vi "M9290A Peak Power.vi"(6 "Reference Level":dbl=20.0, 7 "Route Names":string[](array[string]), 8 "error in":errorcluster, 9 "Span Frequency (50 kHz)":dbl, 10 "Center Frequency (100 MHz)":dbl=1000000000.0, 11 "VISA resource name":refnum<visa-resource-name>="ZVL") -> (0 "error out":errorcluster, 1 "Marker Position":dbl, 2 "Marker Amplitude (Cal)":dbl, 3 "Marker Amplitude (Raw)":dbl)   [LabVIEW 2015]
uses:
  <instrlib>/Agilent MXA Series/Public/Configure/Configure Frequency (Center Span).vi
  <instrlib>/Agilent MXA Series/Public/Configure/Trigger/Configure Trigger (Normal).vi
panel:
  out "VISA resource name out":refnum<visa-resource-name>
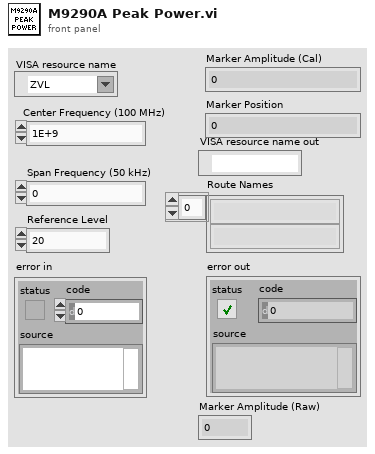
[diagram p1: front panel]
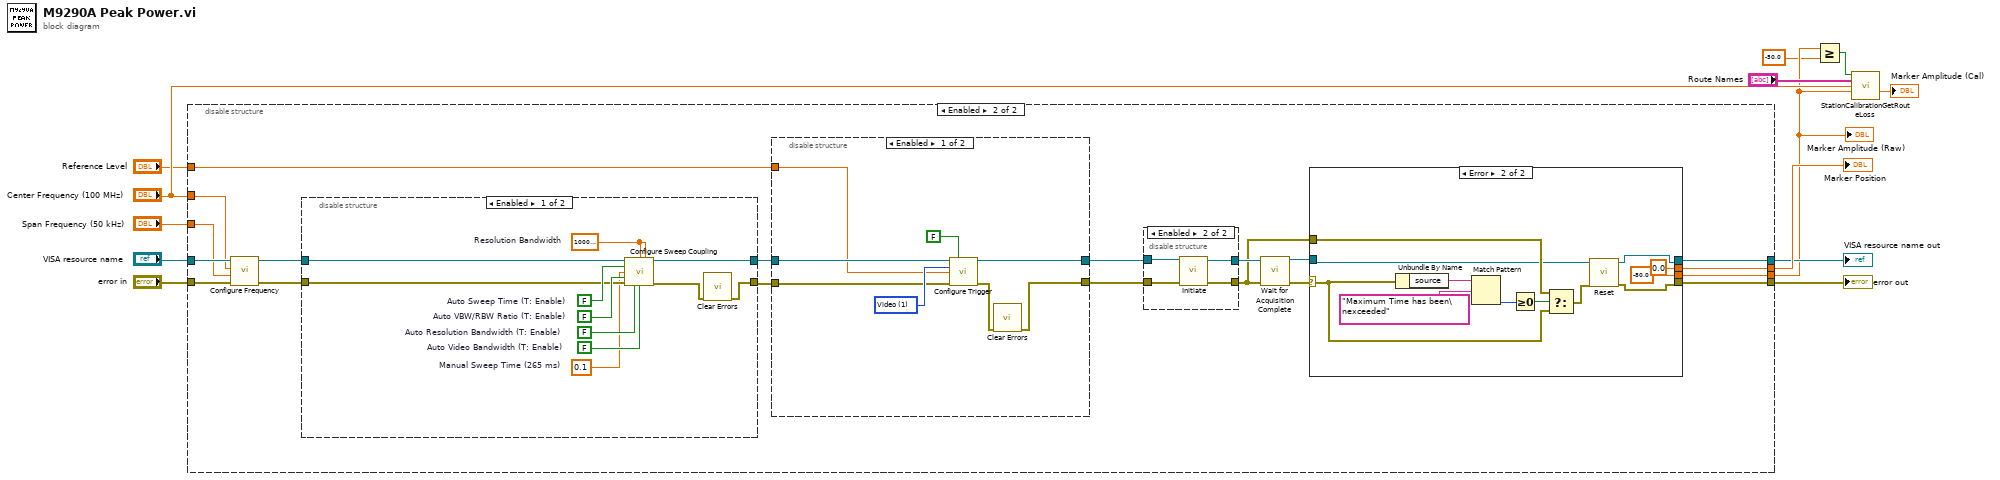
[diagram p0: block diagram]
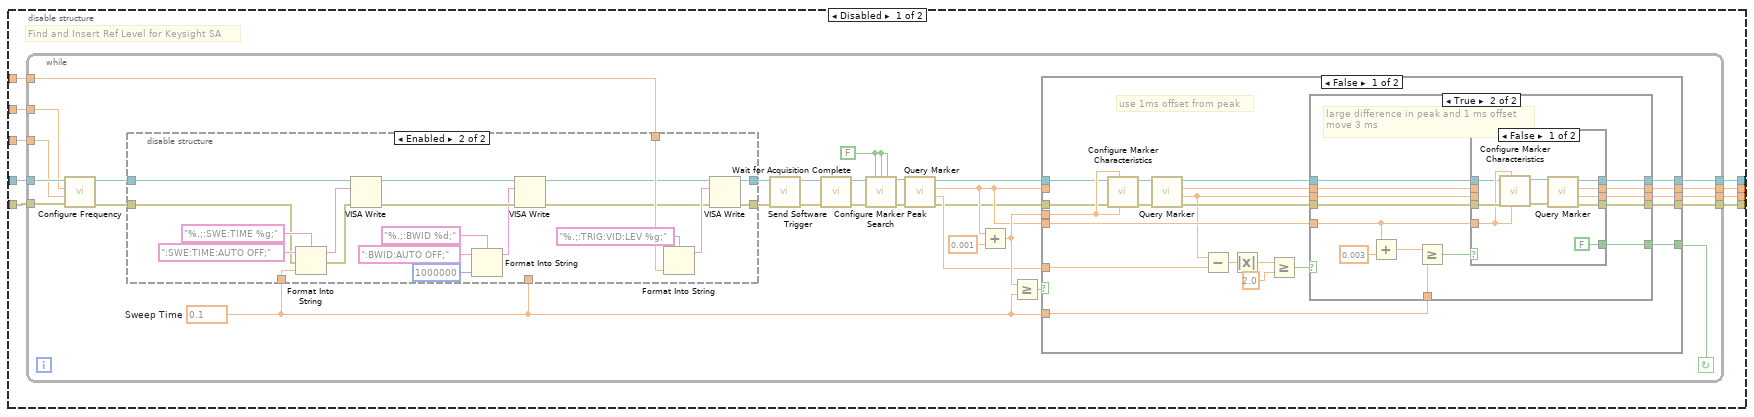
[diagram p2: hidden frame]
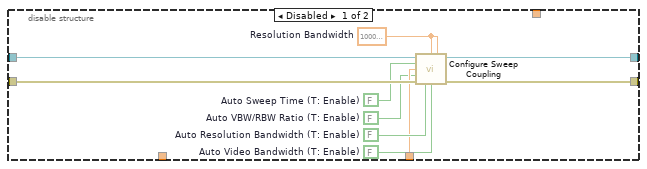
[diagram p3: hidden frame]
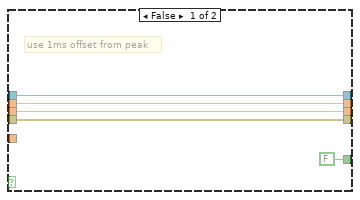
[diagram p4: hidden frame]
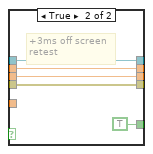
[diagram p5: hidden frame]
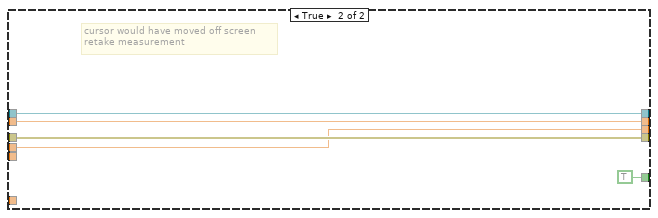
[diagram p6: hidden frame]
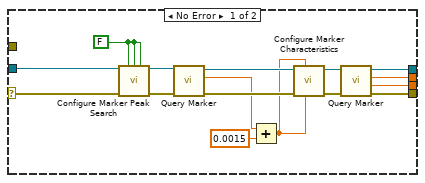
[diagram p7: hidden frame]
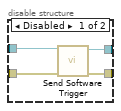
[diagram p8: hidden frame]
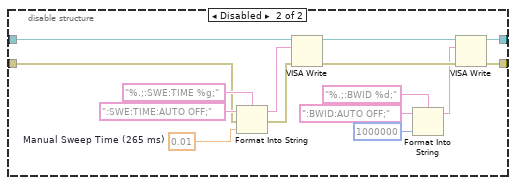
[diagram p10: hidden frame]
diagram:
  n1 = disable-structure shown="Enabled" {
    disable-tunnel: [w22 w151] -> w13
    disable-tunnel: [w21 w154] -> w12
    disable-tunnel: [w20 w153] -> w11
    disable-tunnel: [w19 w152] -> w3
    disable-tunnel: "VISA resource name" -> [w18 w158]
    disable-tunnel: "error in" -> [w17 w157]
    disable-tunnel: "Center Frequency (100 MHz)" -> [w16 w156]
    disable-tunnel: "Span Frequency (50 kHz)" -> [w15 w155]
    disable-tunnel: "Reference Level" -> [w14 w147]
    frame Disabled {
      # "Find and Insert Ref Level for Keysight SA"
      n2 = while {
        tunnel: [w50] -> w21
        tunnel: [w49] -> w19
        tunnel: [w48] -> w22
        tunnel: [w47] -> w20
        tunnel: w18 -> [w28]
        tunnel: w17 -> [w27]
        tunnel: w16 -> [w26]
        tunnel: w15 -> [w25]
        tunnel: w14 -> [w23]
        stop <- w45 continue-if-true
        w24 = 0.1  # Sweep Time
        w33 = FALSE ("Enable Peak Excursion (T: Enable)")
        n3 = call-poly <instrlib>:"Configure Frequency.vi"("error in (no error)"=w27, "Span (2.65E+10 Hz)"=w25, "Center Frequency (1.325E+10 Hz)"=w26, "VISA resource name"=w28) -> ("error out"=w32:errorcluster, "VISA resource name out"=w31:refnum<visa-resource-name>)  [unwired: 6 in]
        n4 = disable-structure shown="Enabled" {
          disable-tunnel: w32 -> [w61 w70]
          disable-tunnel: w31 -> [w60 w71]
          disable-tunnel: [w57 w63] -> w30
          disable-tunnel: [w56 w64] -> w29
          disable-tunnel: w24 -> [w55 _]
          disable-tunnel: w24 -> [_ w69]
          disable-tunnel: w23 -> [_ w66]
          frame Disabled {
            w52 = FALSE  # Auto VBW/RBW Ratio (T: Enable)
            w53 = FALSE  # Auto Video Bandwidth (T: Enable)
            w59 = FALSE  # Auto Sweep Time (T: Enable)
            w58 = FALSE  # Auto Resolution Bandwidth (T: Enable)
            w54 = 1000000.0  # Resolution Bandwidth
            n5 = call <instrlib>:"Configure Sweep Coupling.vi"("VISA resource name"=w60, "Manual Resolution Bandwidth (3E+6 Hz)"=w54, "Manual Video Bandwidth (3E+6 Hz)"=w54, "Auto Sweep Time (T: Enable)"=w59, "Manual Sweep Time (0.0663 s)"=w55, "Auto VBW/RBW Ratio (T: Enable)"=w52, "error in (no error)"=w61, "Auto Resolution Bandwidth (T: Enable)"=w58, "Auto Video Bandwidth (T: Enable)"=w53) -> ("VISA resource name out"=w56:refnum<visa-resource-name>, "error out"=w57:errorcluster)  [unwired: 5 in]
          }
          frame Enabled {
            n6 = Format Into String(format string="%.;:SWE:TIME %g;", initial string=":SWE:TIME:AUTO OFF;", error in=w70, w69) -> (resulting string=w72:string, error out=w73:errorcluster)
            n7 = VISA Write(VISA resource name=w71, write buffer=w72, error in (no error)=w73) -> (VISA resource name out=w81:refnum<visa-resource-name>, error out=w80:errorcluster)  [unwired: 1 out]
            n8 = Format Into String(format string="%.;:BWID %d;", initial string=":BWID:AUTO OFF;" ("format string"), 1000000 ("input 1")) -> (resulting string=w76:string)  [unwired: 1 in, 1 out]
            n9 = VISA Write(VISA resource name=w81, write buffer=w76, error in (no error)=w80) -> (VISA resource name out=w65:refnum<visa-resource-name>, error out=w62:errorcluster)  [unwired: 1 out]
            n10 = Format Into String(format string="%.;:TRIG:VID:LEV %g;", w66) -> (resulting string=w67:string)  [unwired: 2 in, 1 out]
            n11 = VISA Write(VISA resource name=w65, write buffer=w67, error in (no error)=w62) -> (VISA resource name out=w64:refnum<visa-resource-name>, error out=w63:errorcluster)  [unwired: 1 out]
          }
        }
        n12 = call <instrlib>:"Send Software Trigger.vi"("error in (no error)"=w30, "VISA resource name"=w29) -> ("error out"=w42:errorcluster, "VISA resource name out"=w43:refnum<visa-resource-name>)  [unwired: 8 in]
        n13 = call <instrlib>:"Wait for Acquisition Complete.vi"("error in (no error)"=w42, "VISA resource name"=w43) -> ("error out"=w35:errorcluster, "VISA resource name out"=w37:refnum<visa-resource-name>)  [unwired: 8 in]
        n14 = call <instrlib>:"Configure Marker Peak Search.vi"("VISA resource name"=w37, "Enable Peak Excursion (T: Enable)"=w33, "Enable Peak Threshold (T: Enable)"=w33, "Enable Continuous Peak Search (F: Disable)"=w33, "error in (no error)"=w35) -> ("VISA resource name out"=w40:refnum<visa-resource-name>, "error out"=w41:errorcluster)  [unwired: 9 in]
        n15 = call <instrlib>:"Query Marker.vi"("error in (no error)"=w41, "VISA resource name"=w40) -> ("error out"=w34:errorcluster, "Marker Amplitude"=w39:dbl, "Marker Position"=w38:dbl, "VISA resource name out"=w36:refnum<visa-resource-name>)  [unwired: 6 in]
        n16 = Add(x=w38, y=0.001 ("x")) -> (x+y=w44:dbl)
        n17 = Greater Or Equal?(x=w44, y=w24) -> (x >= y?=w46:bool)
        n18 = case shown="False" w46 {
          tunnel: w34 -> [w82 w140]
          tunnel: w36 -> [w85 w141]
          tunnel: w39 -> [w102 _]
          tunnel: w38 -> [w92 _]
          tunnel: [w97 w140] -> w50
          tunnel: [w96 w138] -> w49
          tunnel: [w95 w139] -> w48
          tunnel: [w94 w141] -> w47
          tunnel: w44 -> [w86 w138]
          tunnel: w38 -> [_ w139]
          tunnel: w24 -> [w93 _]
          tunnel: [w91 TRUE] -> w45
          frame False {
            # "use 1ms offset from peak"
            n19 = call <instrlib>:"Configure Marker Characteristics.vi"("Band Right Edge Frequency (0 Hz)"=w86, "Band Left Edge Frequency (0 Hz)"=w86, "error in (no error)"=w82, "VISA resource name"=w85) -> ("error out"=w84:errorcluster, "VISA resource name out"=w83:refnum<visa-resource-name>)  [unwired: 6 in]
            n20 = call <instrlib>:"Query Marker.vi"("error in (no error)"=w84, "VISA resource name"=w83) -> ("error out"=w90:errorcluster, "Marker Amplitude"=w89:dbl, "Marker Position"=w88:dbl, "VISA resource name out"=w87:refnum<visa-resource-name>)  [unwired: 6 in]
            n21 = Subtract(x=w89, y=w102) -> (x-y=w98:dbl)
            n22 = Absolute Value(x=w98) -> (abs(x)=w101:dbl)
            n23 = Greater Or Equal?(x=w101, y=2.0) -> (x >= y?=w99:bool)
            n24 = case shown="True" w99 {
              tunnel: w87 -> [w104 w121]
              tunnel: w90 -> [w105 w120]
              tunnel: w92 -> [_ w112]
              tunnel: [w105 w119] -> w97
              tunnel: [w107 w118] -> w96
              tunnel: [w106 w117] -> w95
              tunnel: w89 -> [w107 w109]
              tunnel: w88 -> [w106 w110]
              tunnel: [w104 w116] -> w94
              tunnel: w93 -> [_ w114]
              tunnel: [FALSE w108] -> w91
              frame False {
                # "use 1ms offset from peak"
              }
              frame True {
                # "large difference in peak and 1 ms offset\nmove 3 ms"
                n25 = Add(x=w112, y=0.003) -> (x+y=w111:dbl)
                n26 = Greater Or Equal?(x=w111, y=w114) -> (x >= y?=w115:bool)
                n27 = case shown="False" w115 {
                  tunnel: w121 -> [w124 w136]
                  tunnel: w120 -> [w126 w133]
                  tunnel: w112 -> [w125 _]
                  tunnel: [w130 w133] -> w119
                  tunnel: [w129 w134] -> w118
                  tunnel: [w127 w135] -> w117
                  tunnel: [w128 w136] -> w116
                  tunnel: w110 -> [_ w135]
                  tunnel: w109 -> [_ w134]
                  tunnel: [FALSE TRUE] -> w108
                  frame False {
                    n28 = call <instrlib>:"Configure Marker Characteristics.vi"("Band Right Edge Frequency (0 Hz)"=w125, "Band Left Edge Frequency (0 Hz)"=w125, "error in (no error)"=w126, "VISA resource name"=w124) -> ("error out"=w122:errorcluster, "VISA resource name out"=w123:refnum<visa-resource-name>)  [unwired: 6 in]
                    n29 = call <instrlib>:"Query Marker.vi"("error in (no error)"=w122, "VISA resource name"=w123) -> ("error out"=w130:errorcluster, "Marker Amplitude"=w129:dbl, "Marker Position"=w127:dbl, "VISA resource name out"=w128:refnum<visa-resource-name>)  [unwired: 6 in]
                  }
                  frame True {
                    # "+3ms off screen\nretest"
                  }
                }
              }
            }
          }
          frame True {
            # "cursor would have moved off screen\nretake measurement"
          }
        }
      }
    }
    frame Enabled {
      n30 = call-poly <instrlib>:"Configure Frequency.vi"("error in (no error)"=w157, "Span (2.65E+10 Hz)"=w155, "Center Frequency (1.325E+10 Hz)"=w156, "VISA resource name"=w158) -> ("error out"=w159:errorcluster, "VISA resource name out"=w160:refnum<visa-resource-name>)  [unwired: 6 in]
      n31 = disable-structure shown="Enabled" {
        disable-tunnel: w160 -> [w212 w220]
        disable-tunnel: w159 -> [w211 w219]
        disable-tunnel: [w207 w222] -> w146
        disable-tunnel: [w210 w221] -> w150
        frame Enabled {
          w209 = 0.1  # Manual Sweep Time (265 ms)
          w213 = FALSE  # Auto VBW/RBW Ratio (T: Enable)
          w214 = FALSE  # Auto Video Bandwidth (T: Enable)
          w217 = FALSE  # Auto Sweep Time (T: Enable)
          w216 = FALSE  # Auto Resolution Bandwidth (T: Enable)
          w215 = 1000000.0  # Resolution Bandwidth
          n32 = call <instrlib>:"Configure Sweep Coupling.vi"("VISA resource name"=w212, "Manual Resolution Bandwidth (3E+6 Hz)"=w215, "Manual Video Bandwidth (3E+6 Hz)"=w215, "Auto Sweep Time (T: Enable)"=w217, "Manual Sweep Time (0.0663 s)"=w209, "Auto VBW/RBW Ratio (T: Enable)"=w213, "error in (no error)"=w211, "Auto Resolution Bandwidth (T: Enable)"=w216, "Auto Video Bandwidth (T: Enable)"=w214) -> ("VISA resource name out"=w210:refnum<visa-resource-name>, "error out"=w208:errorcluster)  [unwired: 5 in]
          n33 = call <vilib>:"Clear Errors.vi"("error in (no error)"=w208) -> ("error out"=w207:errorcluster)  [unwired: 5 in, 1 out]
        }
        frame Disabled {
          w218 = 0.01  # Manual Sweep Time (265 ms)
          n34 = Format Into String(format string="%.;:SWE:TIME %g;", initial string=":SWE:TIME:AUTO OFF;", error in=w219, w218) -> (resulting string=w223:string, error out=w224:errorcluster)
          n35 = VISA Write(VISA resource name=w220, write buffer=w223, error in (no error)=w224) -> (VISA resource name out=w232:refnum<visa-resource-name>, error out=w231:errorcluster)  [unwired: 1 out]
          n36 = Format Into String(format string="%.;:BWID %d;", initial string=":BWID:AUTO OFF;" ("format string"), 1000000 ("input 1")) -> (resulting string=w227:string)  [unwired: 1 in, 1 out]
          n37 = VISA Write(VISA resource name=w232, write buffer=w227, error in (no error)=w231) -> (VISA resource name out=w221:refnum<visa-resource-name>, error out=w222:errorcluster)  [unwired: 1 out]
        }
      }
      n38 = disable-structure shown="Enabled" {
        disable-tunnel: w150 -> [w204 w205]
        disable-tunnel: [w202 w205] -> w149
        disable-tunnel: [w198 w206] -> w148
        disable-tunnel: w147 -> [w197 _]
        disable-tunnel: w146 -> [w200 w206]
        frame Enabled {
          w203 = u16 1 items=["Immediate", "Video", "Line", "RF Burst", "TV", "External1", "External2"] ("Trigger Source (0: Immediate)")
          n39 = call-poly <instrlib>:"Configure Trigger.vi"("VISA resource name"=w204, "Enable Trigger Delay (F: Disable)"=FALSE ("Enable Trigger Delay (T: Enable)"), "Trigger Source (0: Free Run)"=w203, "Trigger Level (-20 dBm)"=w197, "error in (no error)"=w200) -> ("VISA resource name out"=w202:refnum<visa-resource-name>, "error out"=w199:errorcluster)  [unwired: 9 in]
          n40 = call <vilib>:"Clear Errors.vi"("error in (no error)"=w199) -> ("error out"=w198:errorcluster)  [unwired: 5 in, 1 out]
        }
        frame Disabled {
        }
      }
      n41 = disable-structure shown="Enabled" {
        disable-tunnel: [w192 w193] -> w145
        disable-tunnel: [w191 w196] -> w142
        disable-tunnel: w149 -> [w190 w194]
        disable-tunnel: w148 -> [w189 w195]
        frame Disabled {
          n42 = call <instrlib>:"Send Software Trigger.vi"("error in (no error)"=w189, "VISA resource name"=w190) -> ("error out"=w191:errorcluster, "VISA resource name out"=w192:refnum<visa-resource-name>)  [unwired: 8 in]
        }
        frame Enabled {
          n43 = call <instrlib>:"Initiate.vi"("error in (no error)"=w195, "VISA resource name"=w194) -> ("error out"=w196:errorcluster, "VISA resource name out"=w193:refnum<visa-resource-name>)  [unwired: 8 in]
        }
      }
      n44 = call <instrlib>:"Wait for Acquisition Complete.vi"("error in (no error)"=w142, "VISA resource name"=w145) -> ("error out"=w143:errorcluster, "VISA resource name out"=w144:refnum<visa-resource-name>)  [unwired: 8 in]
      n45 = case shown="Error" w143 {
        selector: w143 -> [w161 w181]
        tunnel: [w176 w177] -> w154
        tunnel: [w175 w178] -> w153
        tunnel: [w174 -80.0 ("Marker Amplitude")] -> w152
        tunnel: [w173 0.0 ("Marker Position")] -> w151
        tunnel: w144 -> [w169 w179]
        tunnel: w142 -> [_ w182]
        frame No Error {
          w170 = FALSE ("Enable Peak Excursion (T: Enable)")
          n46 = call <instrlib>:"Configure Marker Peak Search.vi"("VISA resource name"=w169, "Enable Peak Excursion (T: Enable)"=w170, "Enable Peak Threshold (T: Enable)"=w170, "Enable Continuous Peak Search (F: Disable)"=w170, "error in (no error)"=w161) -> ("VISA resource name out"=w171:refnum<visa-resource-name>, "error out"=w172:errorcluster)  [unwired: 9 in]
          n47 = call <instrlib>:"Query Marker.vi"("error in (no error)"=w172, "VISA resource name"=w171) -> ("error out"=w168:errorcluster, "Marker Position"=w165:dbl, "VISA resource name out"=w167:refnum<visa-resource-name>)  [unwired: 6 in, 1 out]
          n48 = Add(x=w165, y=0.0015) -> (x+y=w164:dbl)
          n49 = call <instrlib>:"Configure Marker Characteristics.vi"("Band Right Edge Frequency (0 Hz)"=w164, "Band Left Edge Frequency (0 Hz)"=w164, "error in (no error)"=w168, "VISA resource name"=w167) -> ("error out"=w163:errorcluster, "VISA resource name out"=w162:refnum<visa-resource-name>)  [unwired: 6 in]
          n50 = call <instrlib>:"Query Marker.vi"("error in (no error)"=w163, "VISA resource name"=w162) -> ("error out"=w176:errorcluster, "Marker Amplitude"=w174:dbl, "Marker Position"=w173:dbl, "VISA resource name out"=w175:refnum<visa-resource-name>)  [unwired: 6 in]
        }
        frame Error {
          n51 = Unbundle By Name(w181) -> ("source"=w186:string)
          n52 = Match Pattern(string=w186, regular expression="Maximum Time has been\nexceeded") -> (offset past match=w184:i32)  [unwired: 1 in, 3 out]
          n53 = Greater Or Equal To 0?(x=w184) -> (x >= 0?=w183:bool)
          n54 = Select(t=w182, s=w183, f=w181) -> (s? t:f=w180:errorcluster)
          n55 = call <instrlib>:"Reset.vi"("error in (no error)"=w180, "VISA resource name"=w179) -> ("error out"=w177:errorcluster, "VISA resource name out"=w178:refnum<visa-resource-name>)  [unwired: 8 in]
        }
      }
    }
  }
  "error out" <- w12
  "Marker Position" <- w13
  "VISA resource name out" <- w11
  "Marker Amplitude (Raw)" <- w3
  n56 = Greater Or Equal?(x=w3, y=-50.0) -> (x >= y?=w1:bool)
  n57 = call "StationCalibrationGetRouteLoss.vi"("Calibration Enabled"=w1, "Route Names"="Route Names", "Frequency"="Center Frequency (100 MHz)", "Power Level"=w3) -> ("Adjusted Power Level"=→"Marker Amplitude (Cal)":dbl)  [unwired: 8 in, 3 out]
